vi "Read Auto Version Increment_.vi"(8 "error in (no error)":errorcluster, 11 "EXE Build in":refnum<class "LabVIEW Build.lvclass">) -> (0 "error out":errorcluster, 2 "Auto Version Increment?":bool, 3 "EXE Build out":refnum<class "LabVIEW Build.lvclass">)   [LabVIEW 2014, in "LabVIEW Build.lvclass"]
uses:
  LabVIEW Build.lvclass
  LabVIEW Build.lvclass/LabVIEW Build.ctl
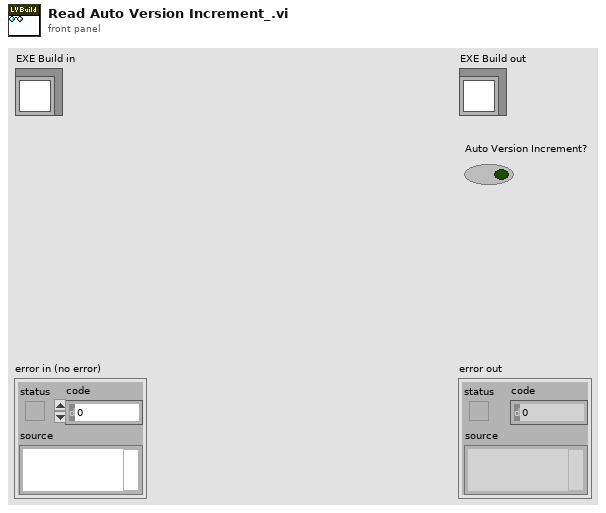
[diagram p1: front panel]
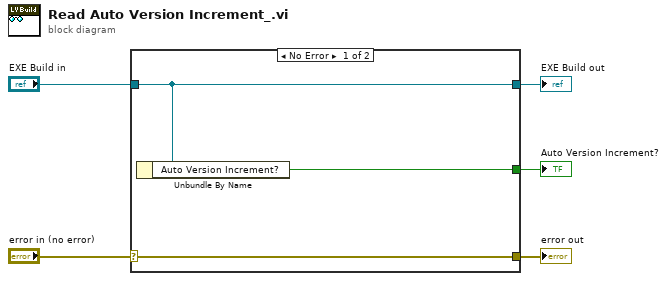
[diagram p0: block diagram]
diagram:
  n1 = case shown="No Error" "error in (no error)" {
    selector: "error in (no error)" -> [w8 w9]
    tunnel: [w8 w9] -> w4
    tunnel: [w7 w10] -> w2
    tunnel: "EXE Build in" -> [w7 w10]
    tunnel: [w6 _] -> w1
    frame No Error {
      n2 = Unbundle By Name(w7) -> ("Auto Version Increment?"=w6:bool)
    }
    frame Error {
    }
  }
  "error out" <- w4
  "EXE Build out" <- w2
  "Auto Version Increment?" <- w1
